vi "HWMatchCheck.vi"(9 "File Mods":string[](array[string]), 11 "Chassis BOM":refnum<class "Chassis BOM.lvclass">) -> (3 "HW Error?":bool)   [LabVIEW 2012, in "Configuration Grandmaster.lvlib" / "Chassis BOM.lvclass"]
uses:
  Chassis BOM.lvclass
  Chassis BOM.lvclass/Chassis BOM.ctl
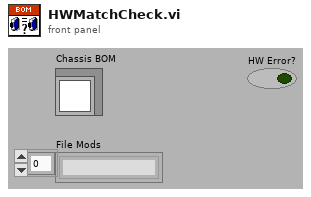
[diagram p1: front panel]
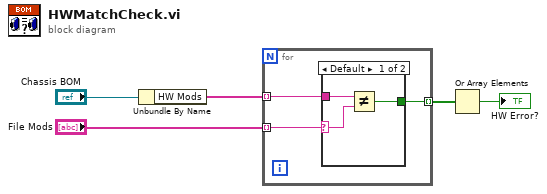
[diagram p0: block diagram]
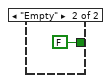
[diagram p2: hidden frame]
diagram:
  n1 = Unbundle By Name("Chassis BOM") -> ("HW Mods"=w3:string[])
  n2 = for {
    tunnel: w3 -> [w7] mode=indexing
    tunnel: "File Mods" -> [w8] mode=indexing
    tunnel: [w6] -> w2 mode=indexing
    n3 = case shown="Default" w8 {
      selector: w8 -> [w10 _]
      tunnel: w7 -> [w11 _]
      tunnel: [w9 FALSE] -> w6
      frame Default {
        n4 = Not Equal?(x=w11, y=w10) -> (x != y?=w9:bool)
      }
      frame "Empty" {
      }
    }
  }
  n5 = Or Array Elements(Boolean array=w2) -> (logical OR=→"HW Error?":bool)
